vi "pc_write_file.vi"(1 "error in":errorcluster, 2 "Write Condition":bool, 3 "Base Path":path, 4 "Data":string, 6 "File Name":string) -> (0 "error out":errorcluster)   [LabVIEW 2013]
doc: "Write data string to a file."
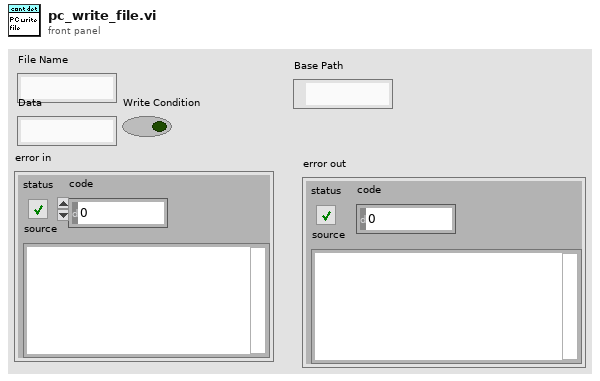
[diagram p1: front panel]
types:
  T1 = enum16{"open", "replace", "create", "open or create", "replace or create", "replace or create with confirmation"}
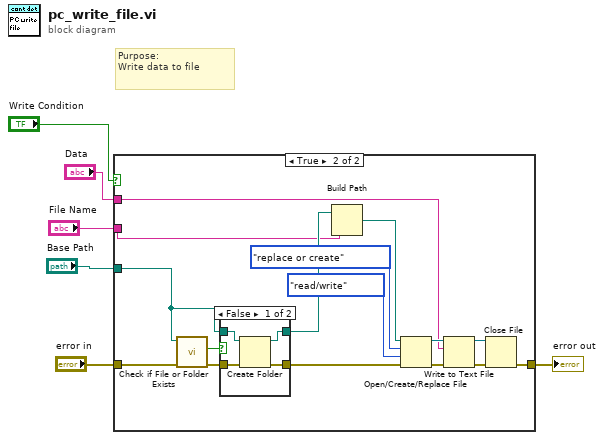
[diagram p0: block diagram]
diagram:
  # "Purpose:\nWrite data to file"
  n1 = case shown="True" "Write Condition" {
    tunnel: "Data" -> [_ w14]
    tunnel: "File Name" -> [_ w11]
    tunnel: "Base Path" -> [_ w8]
    tunnel: [w7 w10] -> w2
    tunnel: "error in" -> [w7 w9]
    frame False {
    }
    frame True {
      n2 = call <vilib>:"Check if File or Folder Exists.vi"("error in (no error)"=w9, "path"=w8) -> ("error out"=w20:errorcluster, "file or folder exists?"=w18:bool)  [unwired: 7 in, 1 out]
      n3 = case shown="False" w18 {
        tunnel: w8 -> [w27 w29]
        tunnel: [w26 w29] -> w17
        tunnel: w20 -> [w25 w28]
        tunnel: [w24 w28] -> w21
        frame False {
          n4 = Create Folder(path (use dialog)=w27, error in=w25) -> (created path=w26:path, error out=w24:errorcluster)  [unwired: 1 in, 1 out]
        }
        frame True {
        }
      }
      n5 = Build Path(base path=w17, name or relative path=w11) -> (appended path=w16:path)
      n6 = Open/Create/Replace File(file path (use dialog)=w16, error in=w21, operation (0:open)=T1."replace or create", access (0:read/write)=enum16{"read/write", "read-only", "write-only"}."read/write") -> (refnum out=w23:refnum<file>, error out=w22:errorcluster)  [unwired: 2 in, 1 out]
      n7 = Write to Text File(file (use dialog)=w23, text=w14, error in=w22) -> (refnum out=w13:refnum<file>, error out=w12:errorcluster)  [unwired: 1 in, 1 out]
      n8 = Close File(refnum=w13, error in=w12) -> (error out=w10:errorcluster)  [unwired: 1 out]
    }
  }
  "error out" <- w2
